vi "gpanel_DO_set_physical_chennels_xy.vi"(8 "error in (no error)":errorcluster, 9 "Y Channel":tag, 10 "X Channel":tag, 11 "galvo_panel in":refnum<class "galvo_panel.lvclass">) -> (0 "error out":errorcluster, 3 "galvo_panel out":refnum<class "galvo_panel.lvclass">)   [LabVIEW 2015, in "galvo_panel.lvclass"]
uses:
  galvo_panel.lvclass
  galvo/galvo.lvclass
  UI/panel_class/panel.lvclass
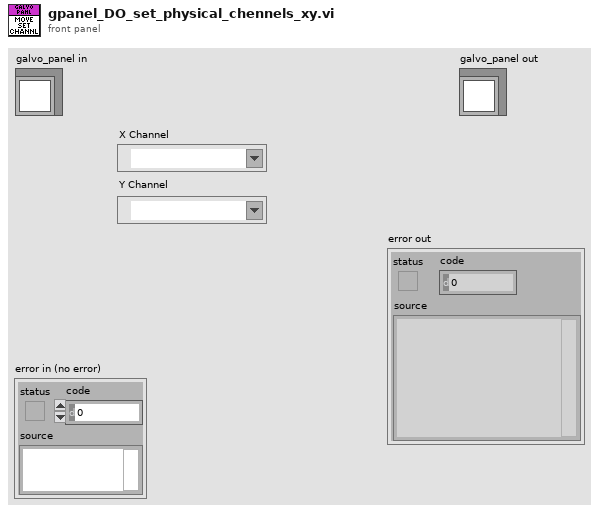
[diagram p1: front panel]
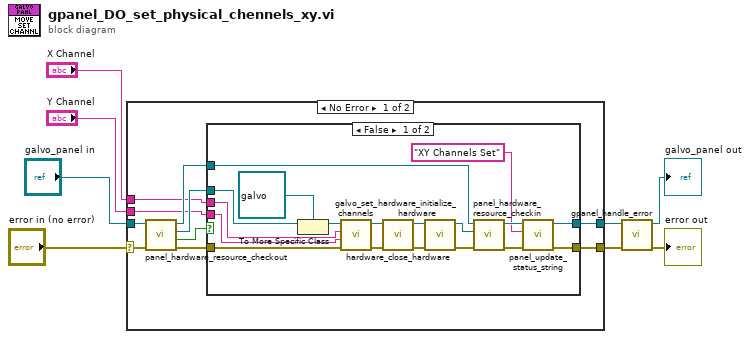
[diagram p0: block diagram]
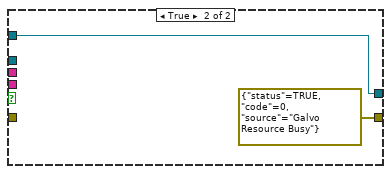
[diagram p2: hidden frame]
diagram:
  n1 = case shown="No Error" "error in (no error)" {
    selector: "error in (no error)" -> [w17 w40]
    tunnel: [w14 w40] -> w3
    tunnel: [w11 w39] -> w4
    tunnel: "galvo_panel in" -> [w18 w39]
    tunnel: "X Channel" -> [w10 _]
    tunnel: "Y Channel" -> [w9 _]
    frame No Error {
      n2 = call "panel_hardware_resource_checkout.vi"("error in (no error)"=w17, "panel in"=w18) -> ("error out"=w15:errorcluster, "timed out?"=w16:bool, "hardware.lvclass"=w13:refnum<class "hardware.lvclass">, "panel out"=w12:refnum<class "galvo_panel.lvclass">)  [unwired: 6 in]
      n3 = case shown="False" w16 {
        tunnel: [w22 errorcluster {"status"=TRUE, "code"=0, "source"="Galvo Resource Busy"} ("error out")] -> w14
        tunnel: w15 -> [w33 _]
        tunnel: w13 -> [w36 _]
        tunnel: w12 -> [w34 w37]
        tunnel: [w21 w37] -> w11
        tunnel: w10 -> [w31 _]
        tunnel: w9 -> [w30 _]
        frame False {
          n4 = To More Specific Class(target class=refnum<class "galvo.lvclass"> refnum ("galvo.lvclass"), reference=w36) -> (specific class reference=w32:refnum<class "galvo.lvclass">)  [unwired: 1 in, 1 out]
          n5 = call "galvo_set_channels.vi"("error in (no error)"=w33, "y_channel"=w30, "x_channel"=w31, "galvo in"=w32) -> ("error out"=w28:errorcluster, "galvo out"=w29:refnum<class "galvo.lvclass">)  [unwired: 6 in]
          n6 = call-dynamic "hardware_close_hardware.vi"("error in (no error)"=w28, "galvo in"=w29) -> ("error out"=w26:errorcluster, "galvo out"=w27:refnum<class "galvo.lvclass">)  [unwired: 8 in]
          n7 = call-dynamic "hardware_initialize_hardware.vi"("error in (no error)"=w26, "galvo in"=w27) -> ("error out"=w24:errorcluster, "galvo out"=w25:refnum<class "galvo.lvclass">)  [unwired: 8 in]
          n8 = call "panel_hardware_resource_checkin.vi"("error in (no error)"=w24, "hardware.lvclass"=w25, "panel in"=w34) -> ("error out"=w23:errorcluster, "panel out"=w20:refnum<class "galvo_panel.lvclass">)  [unwired: 7 in]
          n9 = call-dynamic "panel_update_status_string.vi"("error in (no error)"=w23, "String"="XY Channels Set", "galvo_panel in"=w20) -> ("error out"=w22:errorcluster, "galvo_panel out"=w21:refnum<class "galvo_panel.lvclass">)  [unwired: 7 in]
        }
        frame True {
        }
      }
    }
    frame Error {
    }
  }
  n10 = call "gpanel_handle_error.vi"("error in (no error)"=w3, "galvo_panel in"=w4) -> ("error out"=→"error out":errorcluster, "galvo_panel out"=→"galvo_panel out":refnum<class "galvo_panel.lvclass">)  [unwired: 8 in]
